vi "Start Read Thread.vi"(8 "error in (no error)":errorcluster, 11 "RDS Serial Instrument Actor in":refnum<class "RDS Serial Instrument Actor.lvclass">) -> (0 "error out":errorcluster, 3 "RDS Serial Instrument Actor out":refnum<class "RDS Serial Instrument Actor.lvclass">)   [LabVIEW 2015]
uses:
  Libraries/RDS Serial Handler/RDS Serial Instrument.lvclass
  <vilib>/ActorFramework/Actor/Actor.lvclass
  RDS Serial Instrument Actor Messages/RDS Serial Handle Frame Msg/RDS Serial Handle Frame Msg.lvclass
  RDS Serial Instrument Actor.lvclass
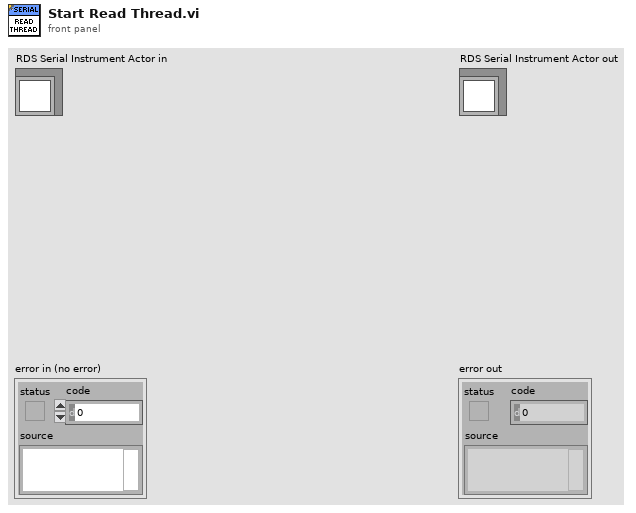
[diagram p1: front panel]
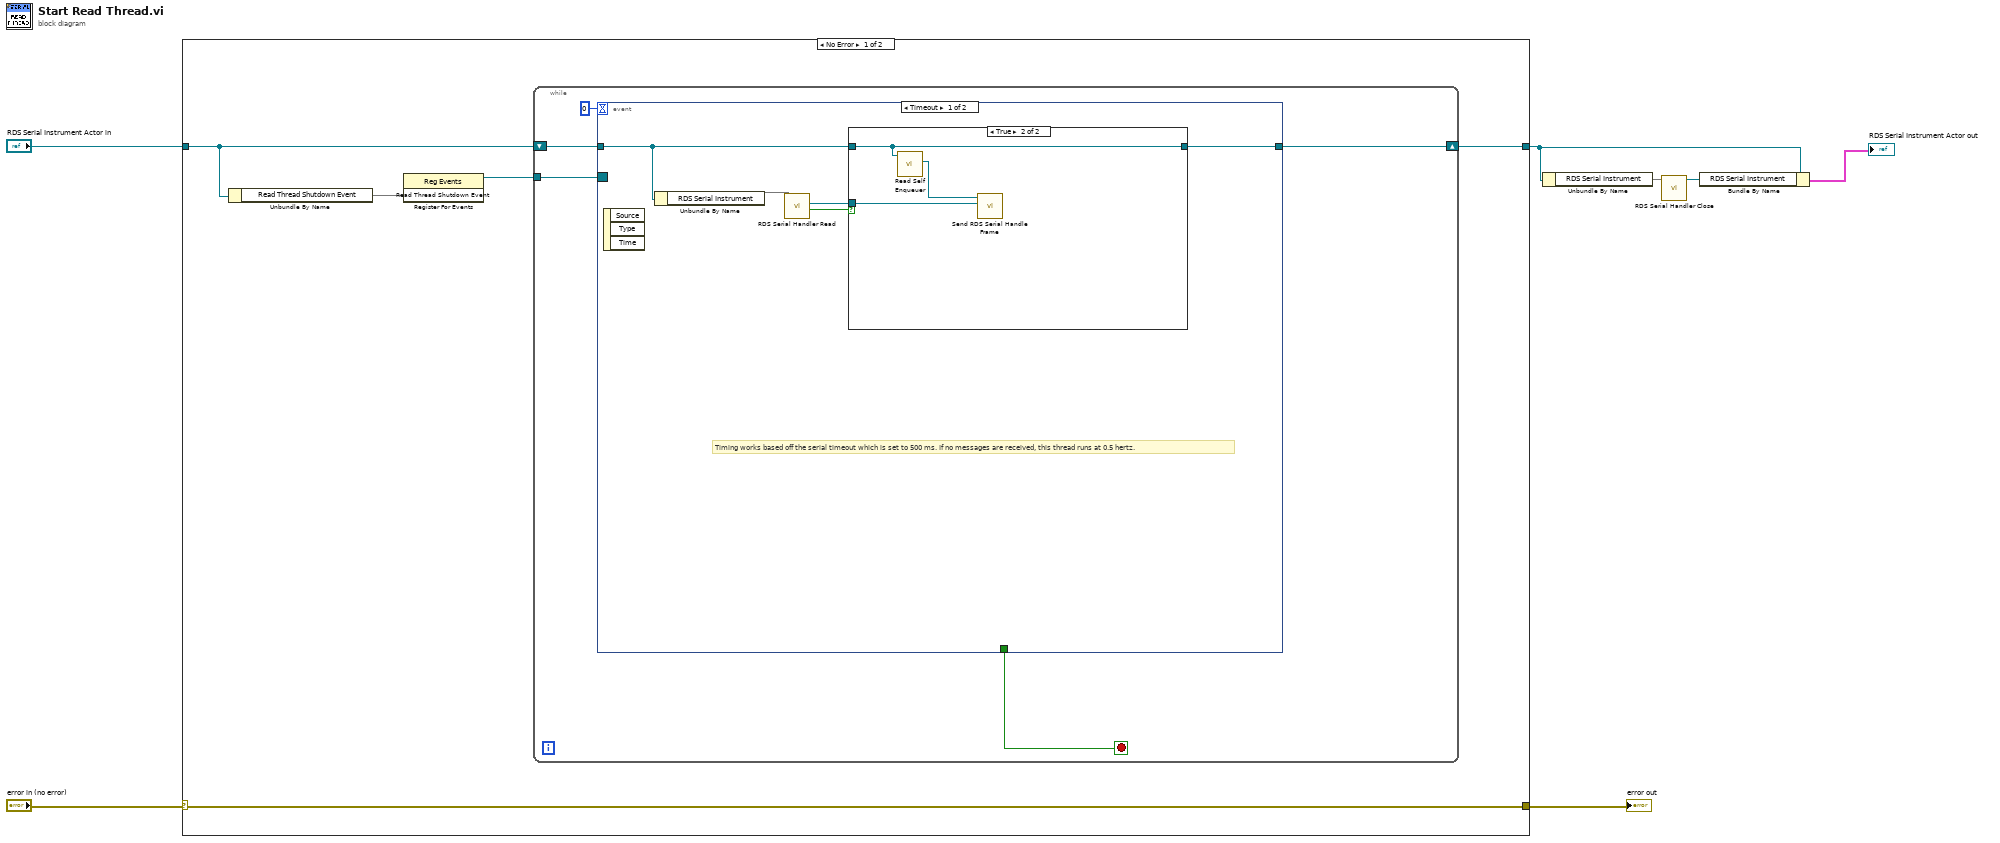
[diagram p0: block diagram]
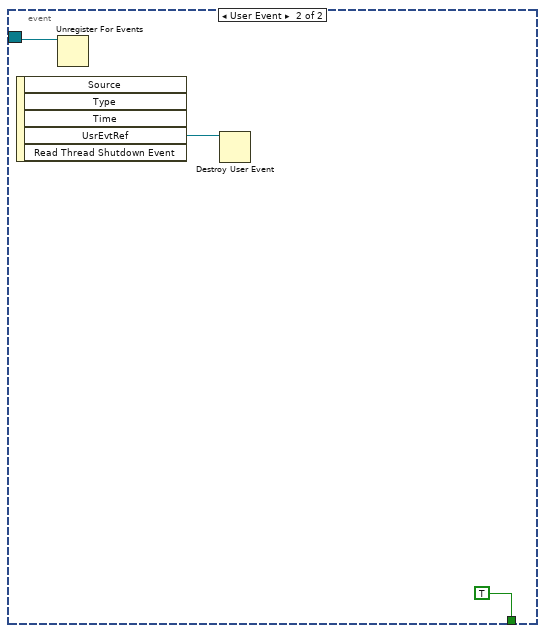
[diagram p3: hidden frame]
diagram:
  n1 = case shown="No Error" "error in (no error)" {
    selector: "error in (no error)" -> [w12 w31]
    tunnel: [w12 w31] -> w6
    tunnel: [w9 w30] -> w2
    tunnel: "RDS Serial Instrument Actor in" -> [w10 w30]
    frame No Error {
      n2 = Unbundle By Name(w10) -> ("Read Thread Shutdown Event"=w11)
      n3 = register-events(w11) -> (reference out=w8:refnum<event-registration>)  [unwired: 2 in, 1 out]
      n4 = while {
        shift-right: [w17] -> w9
        shift-left: w10 -> [w16]
        tunnel: w8 -> [w15]
        stop <- w13 stop-if-true
        n5 = event shown="[0] Timeout" {
          selector: w15 -> [_ w28]
          dyn-events: _ -> [_ _]
          timeout: 0 -> [_ _]
          tunnel: [w21 _] -> w17
          tunnel: w16 -> [w20 _]
          tunnel: [_ TRUE] -> w13
          event Timeout {
            # "Timing works based off the serial timeout which is set to 500 ms. If no messages are received, this thread runs at 0.5 hertz."
            n6 = event-data() -> ()  [unwired: 1 in, 3 out]
            n7 = Unbundle By Name(w20) -> ("RDS Serial Instrument"=w22)
            n8 = call "RDS Serial Handler Read.vi"("RDS Serial Instrument in"=w22) -> ("Data Valid?"=w19:bool, "RDS Serial Frame out"=w18:refnum<class "RDS Serial Frame.lvclass">)  [unwired: 7 in, 2 out]
            n9 = case shown="True" w19 {
              tunnel: [w23 w26] -> w21
              tunnel: w20 -> [w23 w26]
              tunnel: w18 -> [_ w24]
              frame False {
              }
              frame True {
                n10 = call <vilib>:"Read Self Enqueuer.vi"("Actor"=w26) -> ("Self Enqueuer"=w25:refnum<class "Message Enqueuer.lvclass">)  [unwired: 10 in]
                n11 = call "Send RDS Serial Handle Frame.vi"("RDS Serial Frame"=w24, "Message Enqueuer in"=w25) -> ()  [unwired: 8 in, 2 out]
              }
            }
          }
          event User Event {
            n12 = event-data() -> ("UsrEvtRef"=w27:refnum<user-event>)  [unwired: 1 in, 4 out]
            n13 = Unregister For Events(event registration refnum=w28) -> ()  [unwired: 1 in, 1 out]
            n14 = Destroy User Event(user event=w27) -> ()  [unwired: 1 in, 1 out]
          }
        }
      }
    }
    frame Error {
    }
  }
  "error out" <- w6
  n15 = Unbundle By Name(w2) -> ("RDS Serial Instrument"=w4)
  n16 = call "RDS Serial Handler Close.vi"("RDS Serial Instrument in"=w4) -> ("RDS Serial Instrument out"=w3:refnum<class "RDS Serial Instrument.lvclass">)  [unwired: 9 in, 1 out]
  n17 = Bundle By Name(cluster=w2, "RDS Serial Instrument"=w3) -> (→"RDS Serial Instrument Actor out":cluster{})
